vi "Handle Error.vi"(8 "error in (no error)":errorcluster, 11 "UI ActorTop in":refnum<class "UI_Top_Customer.lvclass">) -> (0 "error out":errorcluster, 2 "stop actor?":bool=TRUE, 3 "UI ActorTop out":refnum<class "UI_Top_Customer.lvclass">)   [LabVIEW 2021, in "UI_Top_Customer.lvclass"]
doc: "(<B>Filename</B>: Actor Framework.lvlib:Actor.lvclass:Handle Error.vi)\n\nDefines how the actor handles an error that occurred while processing a message. By default, this method does nothing except stop the actor."
uses:
  UI_Top_Customer.lvclass
  <userlib>/John_Lib/AbstractActorTemplate/AbstractActorTemplate/UIActorTop.lvclass
  UI_Top_Customer.lvclass/UI_Top_Customer.ctl
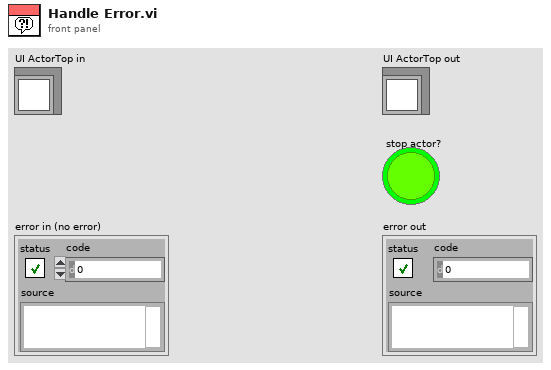
[diagram p1: front panel]
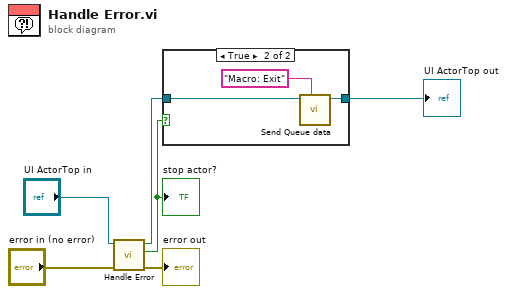
[diagram p0: block diagram]
diagram:
  n1 = call-parent "Handle Error.vi"("error in (no error)"="error in (no error)", "UI ActorTop in"="UI ActorTop in") -> ("error out"=→"error out":errorcluster, "stop actor?"=w3:bool, "UI ActorTop out"=w2:refnum<class "UI_Top_Customer.lvclass">)  [unwired: 7 in]
  "stop actor?" <- w3
  n2 = case shown="True" w3 {
    tunnel: w2 -> [w7 w10]
    tunnel: [w7 w9] -> w1
    frame False {
    }
    frame True {
      n3 = call "Send Queue data.vi"("Elements in Front"="Macro: Exit", "UI_Top_Customer in"=w10) -> ("UI_Top_Customer out"=w9:refnum<class "UI_Top_Customer.lvclass">)  [unwired: 8 in, 1 out]
    }
  }
  "UI ActorTop out" <- w1
